vi "ROS_Master_registerPublisherReply.vi"(2 "PubSub":T2, 3 "ROS_Master in":T1) -> (0 "XML":string)   [LabVIEW 2012]
doc: "Returns XML reply from registering a publisher with the master"
uses:
  <userlib>/ROS for LabVIEW Software/ROS/Code/ROS_Master/ROS_Topic.ctl
  <userlib>/ROS for LabVIEW Software/ROS/Code/ROS_Master/ROS_Master.ctl
  <userlib>/ROS for LabVIEW Software/ROS/Code/ROS_Master/ROS_Node.ctl
  <userlib>/ROS for LabVIEW Software/ROS/Code/ROS_Master/ROS_Service.ctl
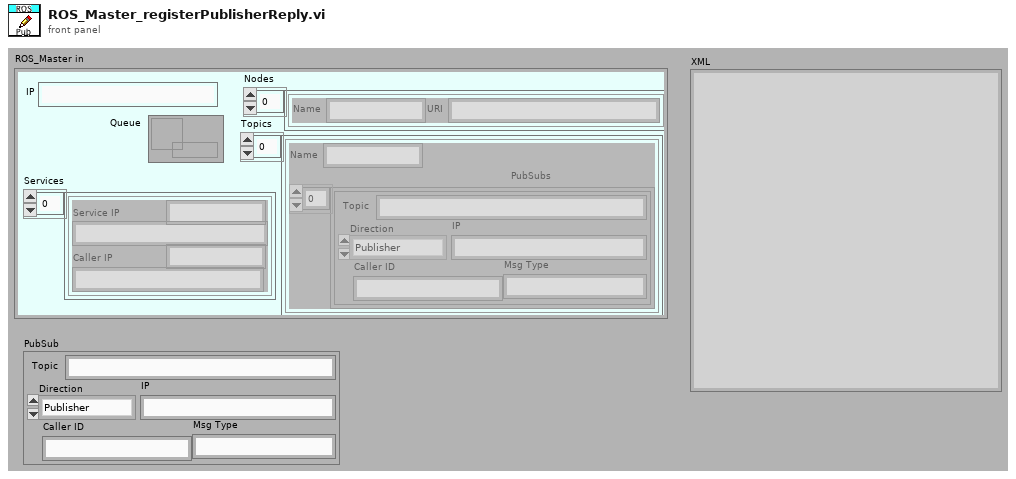
[diagram p1: front panel]
types:
  T1 = typedef "ROS_Master.ctl" = cluster{"IP":string, "Topics":cluster{"Name":string, "PubSubs":T2[]}[], "Nodes":T3[], "Services":T4[], "Queue":refnum<queue>}
  T2 = typedef "ROS_Topic.ctl" = cluster{"Caller ID":string, "IP":string, "Msg Type":string, "Direction":enum16{"Publisher", "Subscriber"}, "Topic":string}
  T3 = typedef "ROS_Node.ctl" = cluster{"Name":string, "URI":string}
  T4 = typedef "ROS_Service.ctl" = cluster{"Service":string, "Service IP":string, "Caller IP":string, "Caller ID":string}
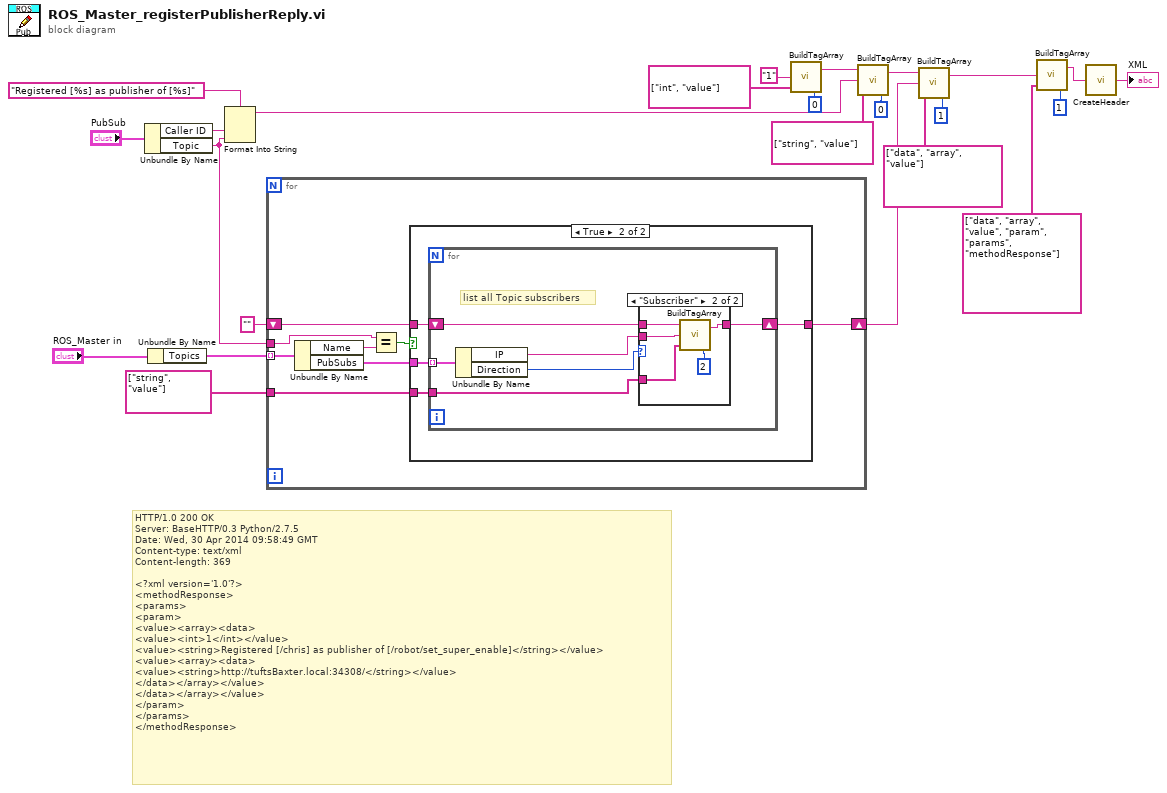
[diagram p0: block diagram]
diagram:
  # "HTTP/1.0 200 OK\nServer: BaseHTTP/0.3 Python/2.7.5\nDate: Wed, 30 Apr 2014 09:58:49 GMT\nContent-type: text/xml\nContent-length: 369\n\n<?xml version='1.0'?>\n<methodResponse>\n<params>\n<param>\n<value><array><data>\n<value><int>1</int></value>\n<value><string>Registered [/chris] as publisher of [/robot/set_super_enable]</string></value>\n<value><array><data>\n<value><string>http://tuftsBaxter.local:34308/</string></value>\n</data></array></value>\n</data></array></value>\n</param>\n</params>\n</methodResponse>"
  n1 = Unbundle By Name("PubSub") -> ("Caller ID"=w19:string, "Topic"=w7:string)
  n2 = Unbundle By Name("ROS_Master in") -> ("Topics"=w24:cluster{"Name":string, "PubSubs":T2[]}[])
  n3 = Format Into String(format string="Registered [%s] as publisher of [%s]", w19, w7) -> (resulting string=w18:string)  [unwired: 2 in, 1 out]
  n4 = for {
    tunnel: w7 -> [w27]
    tunnel: w24 -> [w32] mode=indexing
    shift-right: [w31] -> w22
    shift-left: "" ("string out") -> [w25]
    tunnel: string[] ["string", "value"] ("tags") -> [w29]
    n5 = Unbundle By Name(w32) -> ("Name"=w26:string, "PubSubs"=w30:T2[])
    n6 = Equal?(x=w27, y=w26) -> (x = y?=w28:bool)
    n7 = case shown="True" w28 {
      tunnel: [w33 w37] -> w31
      tunnel: w30 -> [_ w35]
      tunnel: w29 -> [_ w34]
      tunnel: w25 -> [w33 w36]
      frame False {
      }
      frame True {
        n8 = for {
          shift-right: [w43] -> w37
          shift-left: w36 -> [w40]
          tunnel: w35 -> [w42] mode=indexing
          tunnel: w34 -> [w39]
          # "list all Topic subscribers"
          n9 = Unbundle By Name(w42) -> ("IP"=w38:string, "Direction"=w41:enum16{"Publisher", "Subscriber"})
          n10 = case shown="\"Subscriber\"" w41 {
            tunnel: [w44 w49] -> w43
            tunnel: w40 -> [w44 w48]
            tunnel: w39 -> [_ w47]
            tunnel: w38 -> [_ w46]
            frame "Publisher", Default {
            }
            frame "Subscriber" {
              n11 = call <userlib>:"BuildTagArray.vi"("Indent"=i8 2, "tags"=w47, "value"=w46, "string in"=w48) -> ("string out"=w49:string)
            }
          }
        }
      }
    }
  }
  n12 = call <userlib>:"BuildTagArray.vi"("Indent"=i8 0, "tags"=string[] ["int", "value"], "value"="1") -> ("string out"=w14:string)  [unwired: 1 in]
  n13 = call <userlib>:"BuildTagArray.vi"("Indent"=i8 0, "tags"=string[] ["string", "value"], "value"=w18, "string in"=w14) -> ("string out"=w13:string)
  n14 = call <userlib>:"BuildTagArray.vi"("Indent"=i8 1, "tags"=string[] ["data", "array", "value"], "value"=w22, "string in"=w13) -> ("string out"=w12:string)
  n15 = call <userlib>:"BuildTagArray.vi"("Indent"=i8 1, "tags"=string[] ["data", "array", "value", "param", "params", "methodResponse"], "value"=w12) -> ("string out"=w10:string)  [unwired: 1 in]
  n16 = call <userlib>:"CreateHeader.vi"("Content"=w10) -> ("XML"=→"XML":string)
